vi "Unregister Loggers.vi"(8 "error in (no error)":errorcluster) -> (0 "error out":errorcluster, 3 "failures info":T1[](array[typedef]) {"Log Record"."timestamp" format="%<%x %.3X>T"})   [LabVIEW 2018, in "Logging.lvlib"]
uses:
  Logging.lvlib
  Failure Information.ctl
  Log Record.ctl
  Logger/Internal Log Levels.ctl
  Logger/Logger.lvclass
  Registry/Registry.lvlib
panel:
  # "Connector Pane"
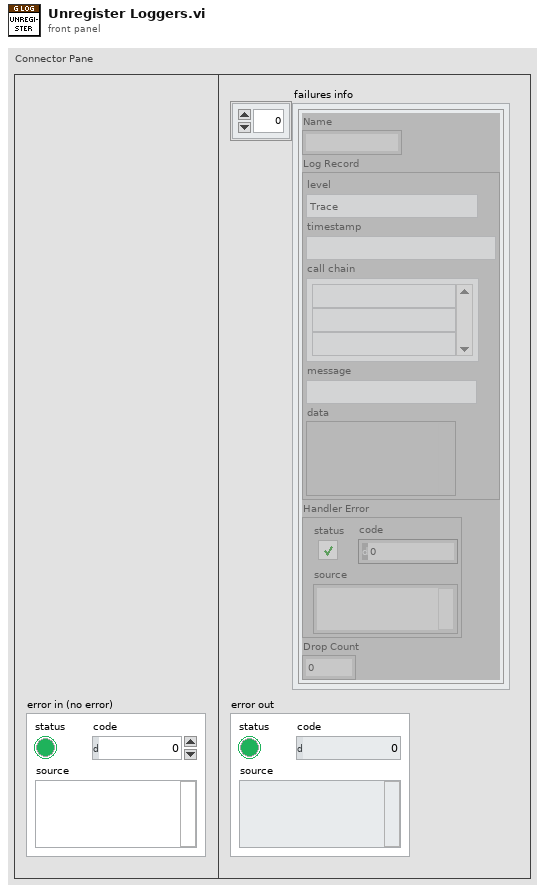
[diagram p1: front panel]
types:
  T1 = typedef "Logging.lvlib/Failure Information.ctl" = cluster{"Name":string, "Log Record":T2, "Handler Error":errorcluster, "Drop Count":u32}
  T2 = typedef "Logging.lvlib/Log Record.ctl" = cluster{"level":T3, "timestamp":timestamp, "call chain":string[], "message":string, "data":variant}
  T3 = typedef "Logging.lvlib/Internal Log Levels.ctl" = enum16{"Trace", "Debug", "Info", "Warning", "Error", "Critical", "Internal"}
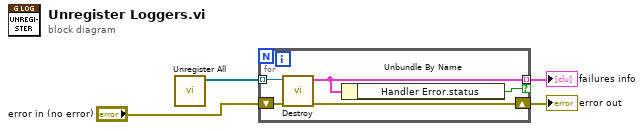
[diagram p0: block diagram]
diagram:
  n1 = call "Unregister All.vi"() -> ("loggers"=w3:refnum<class "Logger.lvclass">[])  [unwired: 11 in]
  n2 = for {
    shift-right: [w8] -> w2
    shift-left: "error in (no error)" -> [w9]
    tunnel: w3 -> [w7] mode=indexing
    tunnel: [w6] -> w4 mode=indexing if=w5
    n3 = call "Destroy.vi"("error in (no error)"=w9, "logger in"=w7) -> ("error out"=w8:errorcluster, "failure info"=w6:T1)  [unwired: 8 in]
    n4 = Unbundle By Name(w6) -> ("Handler Error.status"=w5:bool)
  }
  "failures info" <- w4
  "error out" <- w2
